vi "MGI Save Front Panel Data.vi"(6 "Section Name (\"Data Values\")":string="Data Values", 7 "VI (Caller)":refnum<vi>, 8 "error in (no error)":errorcluster, 11 "Path":path) -> (0 "Error Out":errorcluster)   [LabVIEW 2020]
doc: "Saves the control and indicator data to the specified file in a MGI Read/Write Anything file under the specified section.\nControl and Indicator names must be unique.\n\nAuthored by Shawn Walpole\nsupport@mooregoodideas.com\nwww.mooregoodideas.com\n\nCopyright (c) 2010, Moore Good Ideas, Inc.\n\nAll rights reserved.\n\nRedistribution and use in source and binary forms, with or without modification, are permitted provided that the following conditions are met:\n\n * Redistributions of source code must retain the above copyright notice, this list of conditions and the following disclaimer.\n * Redistributions in binary form must reproduce the above copyright notice, this list of conditions and the following disclaimer in the documentation and/or other materials provided with the distribution.\n * Neither the name of Moore Good Ideas, Inc. nor the names of its contributors may be used to endorse or promote products derived from this software without specific prior written permission.\n\nTHIS SOFTWARE IS PROVIDED BY THE COPYRIGHT HOLDERS AND CONTRIBUTORS \"AS IS\" AND ANY EXPRESS OR IMPLIED WARRANTIES, INCLUDING, BUT NOT LIMITED TO, THE IMPLIED WARRANTIES OF MERCHANTABILITY AND FITNESS FOR A PARTICULAR PURPOSE ARE DISCLAIMED. IN NO EVENT SHALL THE COPYRIGHT OWNER OR CONTRIBUTORS BE LIABLE FOR ANY DIRECT, INDIRECT, INCIDENTAL, SPECIAL, EXEMPLARY, OR CONSEQUENTIAL DAMAGES (INCLUDING, BUT NOT LIMITED TO, PROCUREMENT OF SUBSTITUTE GOODS OR SERVICES; LOSS OF USE, DATA, OR PROFITS; OR BUSINESS INTERRUPTION) HOWEVER CAUSED AND ON ANY THEORY OF LIABILITY, WHETHER IN CONTRACT, STRICT LIABILITY, OR TORT (INCLUDING NEGLIGENCE OR OTHERWISE) ARISING IN ANY WAY OUT OF THE USE OF THIS SOFTWARE, EVEN IF ADVISED OF THE POSSIBILITY OF SUCH DAMAGE."
uses:
  <userlib>/_MGI/Application Control/MGI VI Reference/MGI Caller's VI Reference.vi
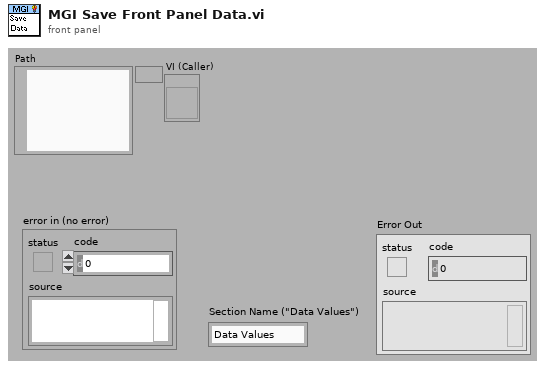
[diagram p1: front panel]
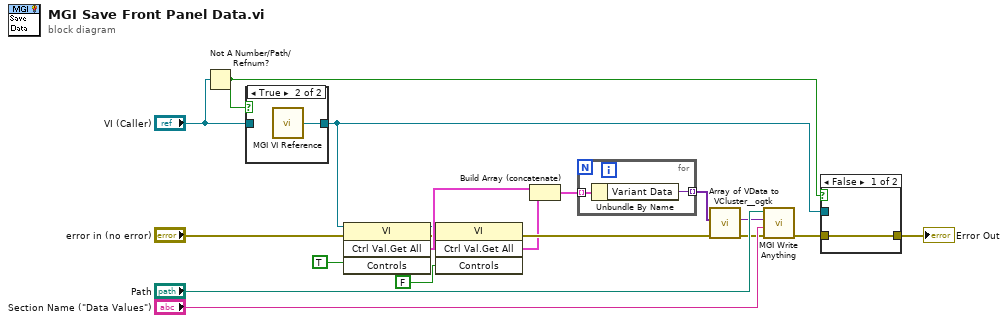
[diagram p0: block diagram]
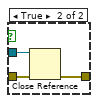
[diagram p2: hidden frame]
diagram:
  n1 = Not A Number/Path/Refnum?(number/path/refnum="VI (Caller)") -> (NaN/Path/Refnum?=w9:bool)
  n2 = case shown="True" w9 {
    tunnel: [w20 w21] -> w17
    tunnel: "VI (Caller)" -> [w20 _]
    frame False {
    }
    frame True {
      n3 = call-poly <userlib>:"MGI VI Reference.vi"() -> ("Caller's VI Reference"=w21:refnum<vi>)  [unwired: 1 in]
    }
  }
  n4 = invoke class="VI" method="Ctrl Val.Get All"(reference=w17, error in="error in (no error)", "Controls"=TRUE) -> (reference out=w12:refnum<vi>, error out=w13:errorcluster, "Get All Control Values Variant"=w14:cluster{"Name":string, "Variant Data":variant}[])  [unwired: 1 in, 1 out]
  n5 = invoke class="VI" method="Ctrl Val.Get All"(reference=w12, error in=w13, "Controls"=FALSE) -> (error out=w18:errorcluster, "Get All Control Values Variant"=w15:cluster{"Name":string, "Variant Data":variant}[])  [unwired: 1 in, 2 out]
  n6 = Build Array (concatenate)(w14, w15) -> (w19:cluster{"Name":string, "Variant Data":variant}[])
  n7 = for {
    tunnel: w19 -> [w23] mode=indexing
    tunnel: [w22] -> w1 mode=indexing
    n8 = Unbundle By Name(w23) -> ("Variant Data"=w22:variant)
  }
  n9 = call <userlib>:"Array of VData to VCluster__ogtk.vi"("error in (no error)"=w18, "Array"=w1) -> ("error out"=w2:errorcluster, "VCluster"=w3:variant)  [unwired: 8 in]
  n10 = call <userlib>:"MGI Write Anything.vi"("Error In"=w2, "Section Name (Name of \"Anything\")"="Section Name (\"Data Values\")", "Anything"=w3, "Path (dialog)"="Path") -> ("Error Out"=w10:errorcluster)  [unwired: 5 in, 2 out]
  n11 = case shown="False" w9 {
    tunnel: w17 -> [_ w27]
    tunnel: w10 -> [w24 w26]
    tunnel: [w24 w25] -> w4
    frame False {
    }
    frame True {
      n12 = Close Reference(reference=w27, error in (no error)=w26) -> (error out=w25:errorcluster)
    }
  }
  "Error Out" <- w4
